vi "Test File Write.vi"() -> ()   [LabVIEW 2014]
uses:
  File.lvclass
  File Class/write bytes.vi
panel:
  out "error out":errorcluster
  in  "error in":errorcluster
  # "There was error with generating writing into file, so this is just to debug\nthis. It has no functionality and it's no DEMO. Maybe in future."
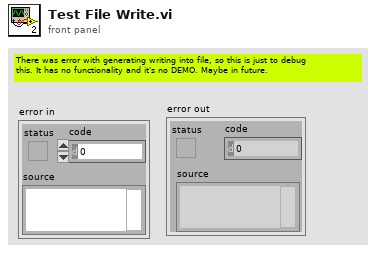
[diagram p1: front panel]
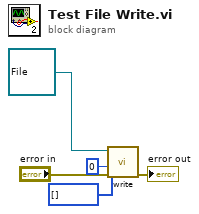
[diagram p0: block diagram]
diagram:
  n1 = call-poly "write.vi"("error in (no error)"="error in", "length"=u32 0, "buffer"=u8[] [], "File in"=refnum<class "File.lvclass"> refnum) -> ("error out"=→"error out":errorcluster)  [unwired: 7 in]
